vi "rqcBob Channel Test (Low Level Example).vi"() -> ()   [LabVIEW 2018]
uses:
  FPGA/rqcBob/Custom Controls/Pulse Train/rqcBob Pulse Train Config.ctl
  FPGA/rqcBob/Custom Controls/Pulse Train/rqcBob Pulse Train.Generation Mode.ctl
  FPGA/rqcBob/Custom Controls/Pulse Train/rqcBob Pulse Train.First Pulse Delay Mode.ctl
  FPGA/rqcBob/Custom Controls/rqcBob Modulator Config.ctl
  FPGA/rqcBob/Custom Controls/rqcBob Window Config.ctl
  Shared/Shared FPGA Lib/Shared Logic/Custom Controls/rqc Random Generator.parameters.ctl
  Shared/Shared FPGA Lib/Shared Logic/Custom Controls/rqc Random Generator.value type.ctl
  FPGA/rqcBob/Custom Controls/rqcBob Trigger Type.ctl
  <vilib>/FPGAPlugInAG/PCIe-7820R/niLvFpga_Open_PCIe-7820R.vi
  <vilib>/rvi/interface/common/dynamic/niFpgaDynamicAddResources.vi
  Low Level API/Configuration/Photon Detector/Detection FIFOs config/rqcBob Configure PD Detect FIFO (1PD PD1).vi
  Low Level API/Read/Read PD Detection FIFO/rqcBob Read PD Detection FIFO (1PD PD1).vi
  <vilib>/FPGAPlugInAG/Dynamic/niLvFpga_Close_Dynamic.vi
  <vilib>/rvi/interface/nirviOpenFPGA/nirviOpenFPGA.xnode
  FPGA Bitfiles/rqcBob (FPGA) 7820 v 4.0.0.lvbitx
  <vilib>/rvi/interface/nirviCloseFPGA/nirviCloseFPGA.xnode
  <vilib>/Analysis/NI_AALBase.lvlib
panel:
  out "DRC":dbl
  out "sum":i32
  in  "modulator.clock delay":fxp<+,4,4>
  out "Done":bool=TRUE
  in  "train.software trigger":bool
  in  "stop":bool
  out "Histogram Graph":T1(graph)
  in  "rndGen.parameters":T2={"value type"=enum."constant", "constant"=150, "num of levels"=4, "levels values"=[0, 0, 0, 0]}
  in  "window.config":T4={"window.open"=0, "window.close"=3000}
  in  "modulator.config":T5={"modulator.start"=1000, "modulator.stop"=2700}
  out "SPD.max meas length":u32=32000
  in  "train.configuration":T6={"period"=4000, "num of pulses"=1, "mode"=enum."train sequence.single", "num of trains"=4000, "first pulse delay mode"=enum."every train", "first pulse delay"=55}
  # "Bob configuration"
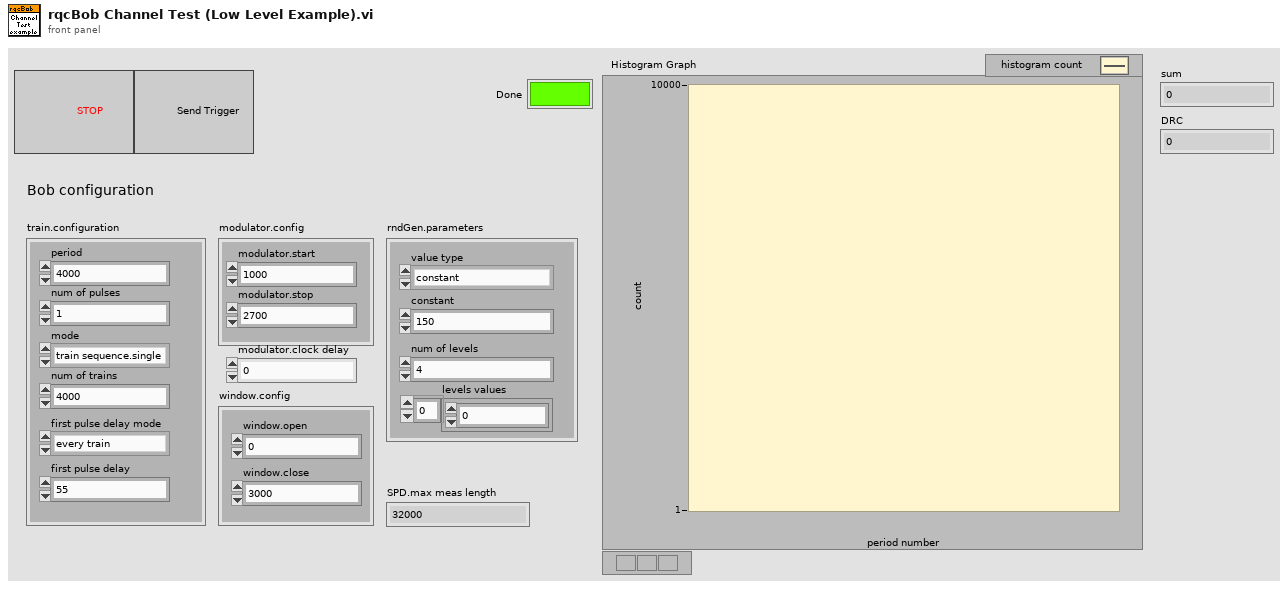
[diagram p1: front panel]
types:
  T1 = cluster{"X Values":dbl[], "Histogram: h(x)":i32[]}
  T2 = typedef "rqc Random Generator.parameters.ctl" = cluster{"value type":T3, "constant":u16, "num of levels":u16, "levels values":u16[]}
  T3 = typedef "rqc Random Generator.value type.ctl" = enum16{"random value", "constant"}
  T4 = typedef "rqcBob Window Config.ctl" = cluster{"window.open":u16, "window.close":u16}
  T5 = typedef "rqcBob Modulator Config.ctl" = cluster{"modulator.start":u16, "modulator.stop":u16}
  T6 = typedef "rqcBob Pulse Train Config.ctl" = cluster{"period":u16, "num of pulses":u16, "mode":T7, "num of trains":u16, "first pulse delay mode":T8, "first pulse delay":u16}
  T7 = typedef "rqcBob Pulse Train.Generation Mode.ctl" = enum8{"single train", "train sequence.single", "train sequence.wait for trigger", "continuous"}
  T8 = typedef "rqcBob Pulse Train.First Pulse Delay Mode.ctl" = enum8{"none", "every train", "first train"}
  T9 = typedef "rqcBob Trigger Type.ctl" = enum16{"software", "immediate", "DIO"}
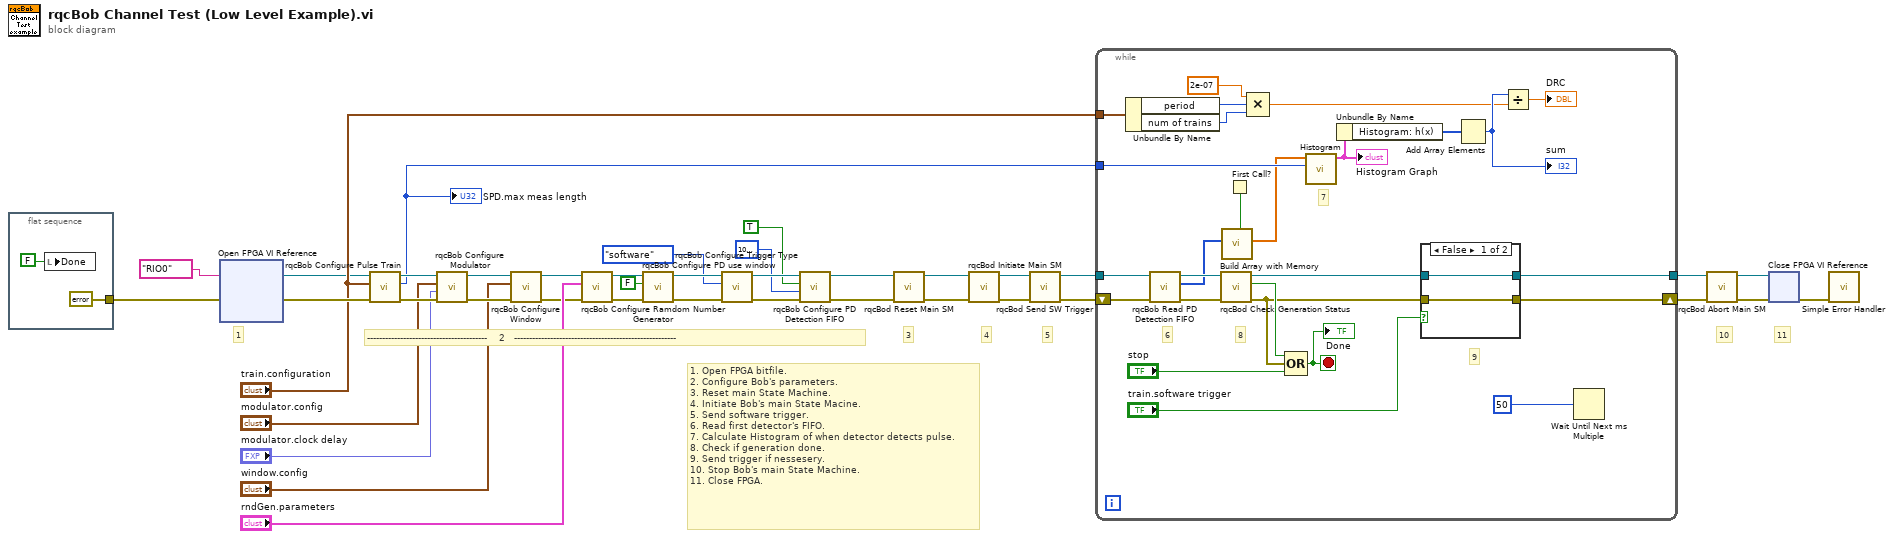
[diagram p0: block diagram]
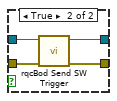
[diagram p2: hidden frame]
diagram:
  # "1. Open FPGA bitfile.\n2. Configure Bob's parameters.\n3. Reset main State Machine.\n4. Initiate Bob's main State Macine.\n5. Send software trigger.\n6. Read first detector's FIFO.\n7. Calculate Histogram of when detector detects pulse.\n8. Check if generation done.\n9. Send trigger if nessesery.\n10. Stop Bob's main State Machine.\n11. Close FPGA."
  # "1"
  # "11"
  # "10"
  # "5"
  # "4"
  # "3"
  # "----------------------------------------    2   ------------------------------------------------------"
  n1 = flat-sequence {
    tunnel: [errorcluster {"status"=FALSE, "code"=0, "source"=""} ("error in")] -> w14
    frame #0 {
      n2 = local write "Done"(FALSE ("Done")) -> ()
    }
  }
  n3 = xnode "Open FPGA VI Reference"("error in"=w14, "resource name"=tag "RIO0") -> ("FPGA VI Reference Out"=w1:refnum<k20>, "error out"=w11:errorcluster)
  n4 = call "rqcBob Configure Pulse Train.vi"("error in"=w11, "train.configuration"="train.configuration", "FPGA reference in"=w1) -> ("error out"=w37:errorcluster, "SPD meas length"=w18:u32, "FPGA reference out"=w38:refnum<k20>)  [unwired: 6 in]
  "SPD.max meas length" <- w18
  n5 = call "rqcBob Configure Modulator.vi"("error in"=w37, "modulator.clock delay"="modulator.clock delay", "modulator.config"="modulator.config", "FPGA reference in"=w38) -> ("error out"=w34:errorcluster, "FPGA reference out"=w35:refnum<k20>)  [unwired: 6 in]
  n6 = call "rqcBob Configure Window.vi"("error in"=w34, "window.config"="window.config", "FPGA reference in"=w35) -> ("error out"=w30:errorcluster, "FPGA reference out"=w31:refnum<k20>)  [unwired: 7 in]
  n7 = call "rqcBob Configure Ramdom Number Generator.vi"("error in"=w30, "rqcBob rndGen.parameters"="rndGen.parameters", "FPGA reference in"=w31) -> ("error out"=w29:errorcluster, "FPGA reference out"=w28:refnum<k20>)  [unwired: 7 in]
  n8 = call "rqcBob Configure PD use window.vi"("error in"=w29, "PD.use window"=FALSE ("SPD.use detector window"), "FPGA reference in"=w28) -> ("error out"=w26:errorcluster, "FPGA reference out"=w27:refnum<k20>)  [unwired: 7 in]
  n9 = call "rqcBob Configure Trigger Type.vi"("error in"=w26, "rqcBob Trigger Type"=rqcBob_Trigger_Type."software", "FPGA reference in"=w27) -> ("error out"=w7:errorcluster, "FPGA reference out"=w9:refnum<k20>)  [unwired: 7 in]
  n10 = call-poly "rqcBob Configure PD Detection FIFO.vi"("error in"=w7, "PD.detect fifo depth"=u32 1000000 ("SPD.detect fifo depth"), "PD.detect fifo write enable"=TRUE ("SPD.detect fifo write enable"), "FPGA reference in"=w9) -> ("error out"=w6:errorcluster, "FPGA reference out"=w8:refnum<k20>)  [unwired: 6 in]
  n11 = call "rqcBod Reset Main SM.vi"("error in"=w6, "FPGA reference in"=w8) -> ("error out"=w23:errorcluster, "FPGA reference out"=w24:refnum<k20>)  [unwired: 8 in]
  n12 = call "rqcBod Initiate Main SM.vi"("error in"=w23, "FPGA reference in"=w24) -> ("error out"=w21:errorcluster, "FPGA reference out"=w22:refnum<k20>)  [unwired: 8 in]
  n13 = call "rqcBod Send SW Trigger.vi"("error in"=w21, "FPGA reference in"=w22) -> ("error out"=w19:errorcluster, "FPGA reference out"=w20:refnum<k20>)  [unwired: 8 in]
  n14 = while {
    tunnel: w20 -> [w56]
    shift-right: [w62] -> w17
    shift-left: w19 -> [w53]
    tunnel: w18 -> [w65]
    tunnel: [w61] -> w3
    tunnel: "train.configuration" -> [w50]
    stop <- w59 stop-if-true
    # "7"
    # "9"
    # "8"
    # "6"
    n15 = Unbundle By Name(w50) -> ("period"=w49:u16, "num of trains"=w47:u16)
    n16 = call-poly "rqcBob Read PD Detection FIFO.vi"("error in"=w53, "FPGA reference in"=w56) -> ("error out"=w52:errorcluster, "Data"=w54:u32[], "FPGA reference out"=w55:refnum<k20>)  [unwired: 6 in, 1 out]
    n17 = call "rqcBod Check Generation Status.vi"("error in"=w52, "FPGA reference in"=w55) -> ("error out"=w63:errorcluster, "generation.done"=w66:bool, "FPGA reference out"=w64:refnum<k20>)  [unwired: 7 in]
    n18 = First Call?() -> (First Call?: T/F=w57:bool)
    n19 = call "Build Array with Memory.vi"("reset"=w57, "new array"=w54) -> ("appended array"=w51:dbl[])  [unwired: 9 in]
    n20 = Compound Arithmetic op=MULTIPLY(2e-07, w49, w47) -> (w43:dbl)
    n21 = Compound Arithmetic op=OR(w66, w63, "stop") -> (w59:bool)
    "Done" <- w59
    n22 = call <vilib>:"Histogram.vi"("intervals"=w65, "X"=w51) -> ("Histogram Graph"=w46:T1)  [unwired: 6 in, 3 out]
    "Histogram Graph" <- w46
    n23 = Unbundle By Name(w46) -> ("Histogram: h(x)"=w45:i32[])
    n24 = case shown="False" "train.software trigger" {
      tunnel: w64 -> [w69 w73]
      tunnel: w63 -> [w68 w72]
      tunnel: [w69 w71] -> w61
      tunnel: [w68 w70] -> w62
      frame False {
      }
      frame True {
        n25 = call "rqcBod Send SW Trigger.vi"("error in"=w72, "FPGA reference in"=w73) -> ("error out"=w70:errorcluster, "FPGA reference out"=w71:refnum<k20>)  [unwired: 8 in]
      }
    }
    n26 = Add Array Elements(numeric array=w45) -> (sum=w44:i32)
    "sum" <- w44
    n27 = Divide(x=w44, y=w43) -> (x/y=→"DRC":dbl)
    n28 = Wait Until Next ms Multiple(millisecond multiple=u32 50) -> ()  [unwired: 1 out]
  }
  n29 = call "rqcBod Abort Main SM.vi"("error in"=w17, "FPGA reference in"=w3) -> ("error out"=w15:errorcluster, "FPGA reference out"=w16:refnum<k20>)  [unwired: 8 in]
  n30 = xnode "Close FPGA VI Reference"("FPGA VI Reference In"=w16, "error in"=w15) -> ("error out"=w13:errorcluster)
  n31 = call <vilib>:"Simple Error Handler.vi"("error in (no error)"=w13) -> ()  [unwired: 4 in, 5 out]
